vi "更新log记录.vi"(7 "路径":path, 8 "错误输入（无错误）":errorcluster, 10 "logname":string, 11 "数组":string[](array[string])) -> (0 "错误输出":errorcluster)   [LabVIEW 2016, in "数据传输系统-06.lvlib" / "自动更新.lvlib"]
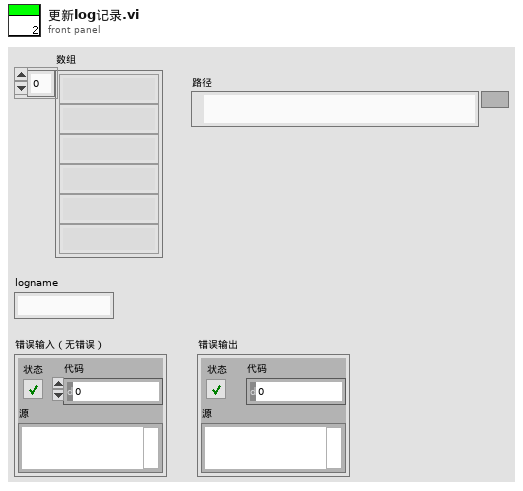
[diagram p1: front panel]
types:
  T1 = enum16{"open", "replace", "create", "open or create", "replace or create", "replace or create with confirmation"}
  T2 = typedef "LVDateTimeRec.ctl" = cluster{"秒数的小数部分":dbl, "秒":i32, "分":i32, "时":i32, "日":i32, "月":i32, "年":i32, "天数（周）":i32, "天数（年）":i32, "DST":i32}
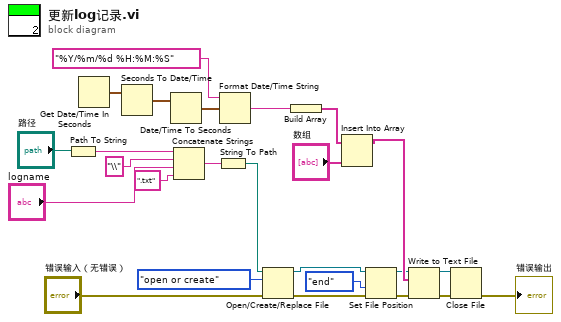
[diagram p0: block diagram]
diagram:
  n1 = Path To String(path="路径") -> (string=w9:string)
  n2 = Get Date/Time In Seconds() -> (seconds since 1Jan1904=w17:timestamp)
  n3 = Seconds To Date/Time(time stamp (now)=w17) -> (date time rec=w20:T2)  [unwired: 1 in]
  n4 = Date/Time To Seconds(2:w20) -> (0:w18:timestamp)  [unwired: 1 in]
  n5 = Concatenate Strings(w9, "\\" ("字符串"), "logname", ".txt" ("字符串")) -> (w7:string)
  n6 = String To Path(string=w7) -> (path=w11:path)
  n7 = Format Date/Time String(time format string (%c)="%Y/%m/%d %H:%M:%S" ("时间格式字符串(%c)"), seconds (now)=w18) -> (date/time string=w21:string)  [unwired: 1 in]
  n8 = Open/Create/Replace File(file path (use dialog)=w11, error in="错误输入（无错误）", operation (0:open)=T1."open or create" ("操作(0:open)")) -> (refnum out=w6:refnum<file>, error out=w5:errorcluster)  [unwired: 3 in, 1 out]
  n9 = Build Array(w21) -> (w16:string[])
  n10 = Insert Into Array(array=w16, new element="数组") -> (w23:string[])  [unwired: 1 in]
  n11 = Set File Position(refnum=w6, from (0:start)=enum16{"start", "end", "current"}."end" ("自（0:起始）"), error in=w5) -> (refnum out=w4:refnum<file>, error out=w3:errorcluster)  [unwired: 1 in]
  n12 = Write to Text File(file (use dialog)=w4, text=w23, error in=w3) -> (refnum out=w12:refnum<file>, error out=w13:errorcluster)  [unwired: 1 in, 1 out]
  n13 = Close File(refnum=w12, error in=w13) -> (error out=→"错误输出":errorcluster)  [unwired: 1 out]
